vi "TDMS Read Property Value (DBL).vi"(2 "Property Name":string, 3 "Property Names":string[](array[string]), 4 "Property Values":variant[](array[variant])) -> (0 "Found?":bool, 1 "Property Value":dbl)   [LabVIEW 2011]
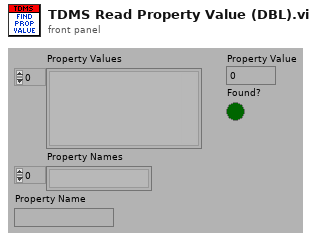
[diagram p1: front panel]
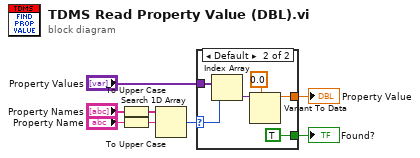
[diagram p0: block diagram]
diagram:
  n1 = To Upper Case(1:"Property Names") -> (0:w6:string[])
  n2 = To Upper Case(1:"Property Name") -> (0:w5:string)
  n3 = Search 1D Array(1D array=w6, element=w5) -> (index of element=w8:i32)  [unwired: 1 out]
  n4 = case shown="Default" w8 {
    selector: w8 -> [_ w13]
    tunnel: "Property Values" -> [_ w14]
    tunnel: [_ w10] -> w7
    tunnel: [_ TRUE ("Found?")] -> w4
    frame -1 {
    }
    frame Default {
      n5 = Index Array(array=w14, index=w13) -> (element=w12:variant)
      n6 = Variant To Data(type=0.0, Variant=w12) -> (data=w10:dbl)  [unwired: 1 in, 1 out]
    }
  }
  "Property Value" <- w7
  "Found?" <- w4
